vi "SVL Scale Voltage to EU (N Ch - N Info).vi"(7 "write waveform attributes? (T)":bool=TRUE, 8 "error in (no error)":errorcluster, 10 "channel info":T1[](array[typedef]) {"pregain" format="%.2f"; "weighting filter" items=["Linear", "A-weighting", "B-weighting", "C-weighting", "ITU-R 468-4", "Dolby", "CCITT", "C-message", "Wb", "Wc", "Wd", "We", "Wf", "Wh", "Wj", "Wk", "Wm", "AES17 20 kHz lowpass", "AES17 40 kHz lowpass", "AES17 20 kHz highpass", "AES17 40 kHz highpass"]; "dB reference" format="%^.1e"; "engineering units" items=["custom..."=0, "V"=1, "A"=21, "C"=30, "pC"=31, "s"=32, "-"=29, "Pa"=2, "N"=20, "g"=3, "m/s^2"=4, "m/s"=5, "m"=6, "mm/s"=12, "mm"=13, "micron/s"=14, "micron"=15, "in/s^2"=7, "in/s"=8, "in"=9, "mil/s"=10, "mil"=11, "rad/s^2"=16, "rad/s"=17, "rad"=18, "deg/s^2"=26, "deg/s"=27, "deg"=28, "RPM"=22, "cycle/s^2"=23, "Hz"=24, "cycle"=25, "strain"=19]; "sensor sensitivity" format="%#_5f"}, 11 "signals [V]":waveform(dbl)[](array[waveform])) -> (0 "error out":errorcluster, 2 "unit labels":string[](array[string]), 3 "scaled signals [EU]":waveform(dbl)[](array[waveform]))   [LabVIEW 2017, in "SoundVib_Calibration.lvlib"]
doc: "Scales <B>signal [V]</B> from volts to the engineering units (EU) you select. Wire data to the <B>signal [V]</B> input to determine the polymorphic instance to use or manually select the instance."
uses:
  <vilib>/addons/Sound and Vibration/svt_Calibration/SoundVib_Calibration.lvlib
  <vilib>/addons/_NISVFA/_Shared subVIs/Controls/svc_Channel Info.ctl
  <vilib>/addons/_NISVFA/_Shared subVIs/Controls/svc_Engineering Units Text Ring.ctl
  <vilib>/addons/_NISVFA/_Shared subVIs/Controls/svc_Weighting Filter Text Ring.ctl
  <vilib>/addons/_NISVFA/_Shared subVIs/Common/svc_Set SV Channel Info.vi
  <vilib>/addons/_NISVFA/_Shared subVIs/Common/svc_Set SV Channel Info (variant).vi
  <vilib>/addons/_NISVFA/_Shared subVIs/Common/SVL Set dB Reference (variant).vi
  <vilib>/addons/_NISVFA/_Shared subVIs/Common/svc_Engineering Units to Unit Label.vi
  <vilib>/addons/_NISVFA/_Shared subVIs/Common/svc_Set dB ref if Pascal.vi
  <vilib>/addons/_NISVFA/_Shared subVIs/Common/svc_Compute Scale Factor to Convert C to EU.vi
  <vilib>/addons/_NISVFA/_Shared subVIs/Common/svc_Compute Scale Factor to Convert V to EU.vi
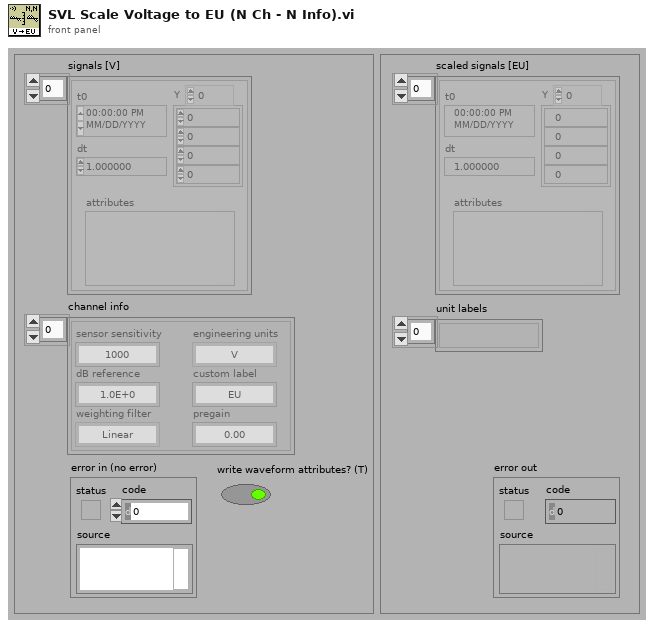
[diagram p1: front panel]
types:
  T1 = typedef "svc_Channel Info.ctl" = cluster{"sensor sensitivity":dbl, "engineering units":T2, "dB reference":dbl, "custom label":string, "weighting filter":T3, "pregain":dbl}
  T2 = typedef "svc_Engineering Units Text Ring.ctl" = u16
  T3 = typedef "svc_Weighting Filter Text Ring.ctl" = u16
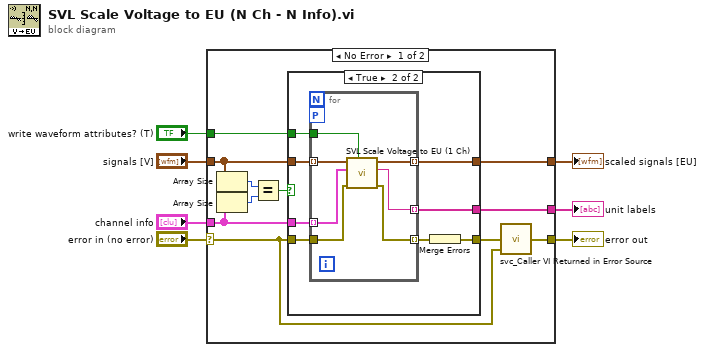
[diagram p0: block diagram]
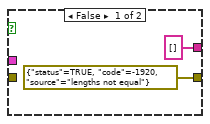
[diagram p2: hidden frame]
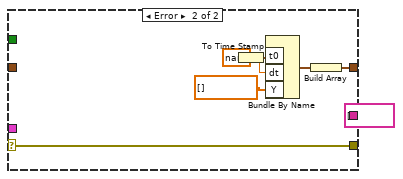
[diagram p3: hidden frame]
diagram:
  n1 = case shown="No Error" "error in (no error)" {
    selector: "error in (no error)" -> [w9 w42]
    tunnel: "signals [V]" -> [w16 _]
    tunnel: "channel info" -> [w15 _]
    tunnel: [w18 w37] -> w7
    tunnel: [w10 w42] -> w6
    tunnel: [w11 string[] []] -> w2
    tunnel: "write waveform attributes? (T)" -> [w8 _]
    frame No Error {
      n2 = Array Size(array=w16) -> (size(s)=w14:i32)
      n3 = Array Size(array=w15) -> (size(s)=w13:i32)
      n4 = Equal?(x=w14, y=w13) -> (x = y?=w12:bool)
      n5 = case shown="True" w12 {
        tunnel: [_ w28] -> w18
        tunnel: [errorcluster {"status"=TRUE, "code"=-1920, "source"="lengths not equal"} ("error out") w21] -> w17
        tunnel: w9 -> [_ w26]
        tunnel: w16 -> [_ w25]
        tunnel: w15 -> [_ w24]
        tunnel: [string[] [] w23] -> w11
        tunnel: w8 -> [_ w22]
        frame False {
        }
        frame True {
          n6 = for {
            tunnel: w25 -> [w35] mode=indexing
            tunnel: w24 -> [w34] mode=indexing
            tunnel: [w32] -> w28 mode=indexing
            tunnel: [w31] -> w23 mode=indexing
            tunnel: w22 -> [w30]
            workers-P: _ -> [_]
            tunnel: w26 -> [w33]
            tunnel: [w29] -> w27 mode=indexing
            n7 = call <vilib>:"SVL Scale Voltage to EU (1 Ch).vi"("write waveform attributes? (T)"=w30, "error in (no error)"=w33, "channel info"=w34, "signal [V]"=w35) -> ("error out"=w29:errorcluster, "unit label"=w31:string, "scaled signal [EU]"=w32:waveform(dbl))  [unwired: 5 in]
          }
          n8 = Merge Errors(w27) -> (w21:errorcluster)
        }
      }
      n9 = call <vilib>:"svc_Caller VI Returned in Error Source.vi"("warning input to caller"=w9, "error in (no error)"=w17) -> ("error out"=w10:errorcluster)  [unwired: 3 in]
    }
    frame Error {
      w40 = nan ("t0")
      n10 = To Time Stamp(1:w40) -> (0:w36:timestamp)
      n11 = Bundle By Name("t0"=w36, "dt"=w40, "Y"=dbl[] []) -> (w38:waveform(dbl))  [unwired: 1 in]
      n12 = Build Array(w38) -> (w37:waveform(dbl)[])
    }
  }
  "scaled signals [EU]" <- w7
  "error out" <- w6
  "unit labels" <- w2
